vi "Display_data.vi"() -> ()   [LabVIEW 2016]
uses:
  <vilib>/Utility/file.llb/Read Delimited Spreadsheet (DBL).vi
panel:
  in  "Boolean":bool
  in  "STOP ALL":bool
  in  "stop":bool
  in  "Ring":u16(ring) items=["Default", "Number Filter", "Average", "Integrate", "Derivate", "g"]
  in  "String":string
  out "Waveform Graph 2":dbl[](graph)
  out "Array":dbl[](array[numeric])
  in  "X vector":i32
  out "XY Graph":cluster{dbl[], "all rows":dbl[]}[](graph)
  in  "Inoput":dbl=15.0 format="%#_13g"
  in  "index (row) 3":i32
  in  "index (row) 2":i32
  in  "index (row)":i32
  out "all rows":dbl[][](array[numeric])
  out "Raw Data":dynamicdata(graph)
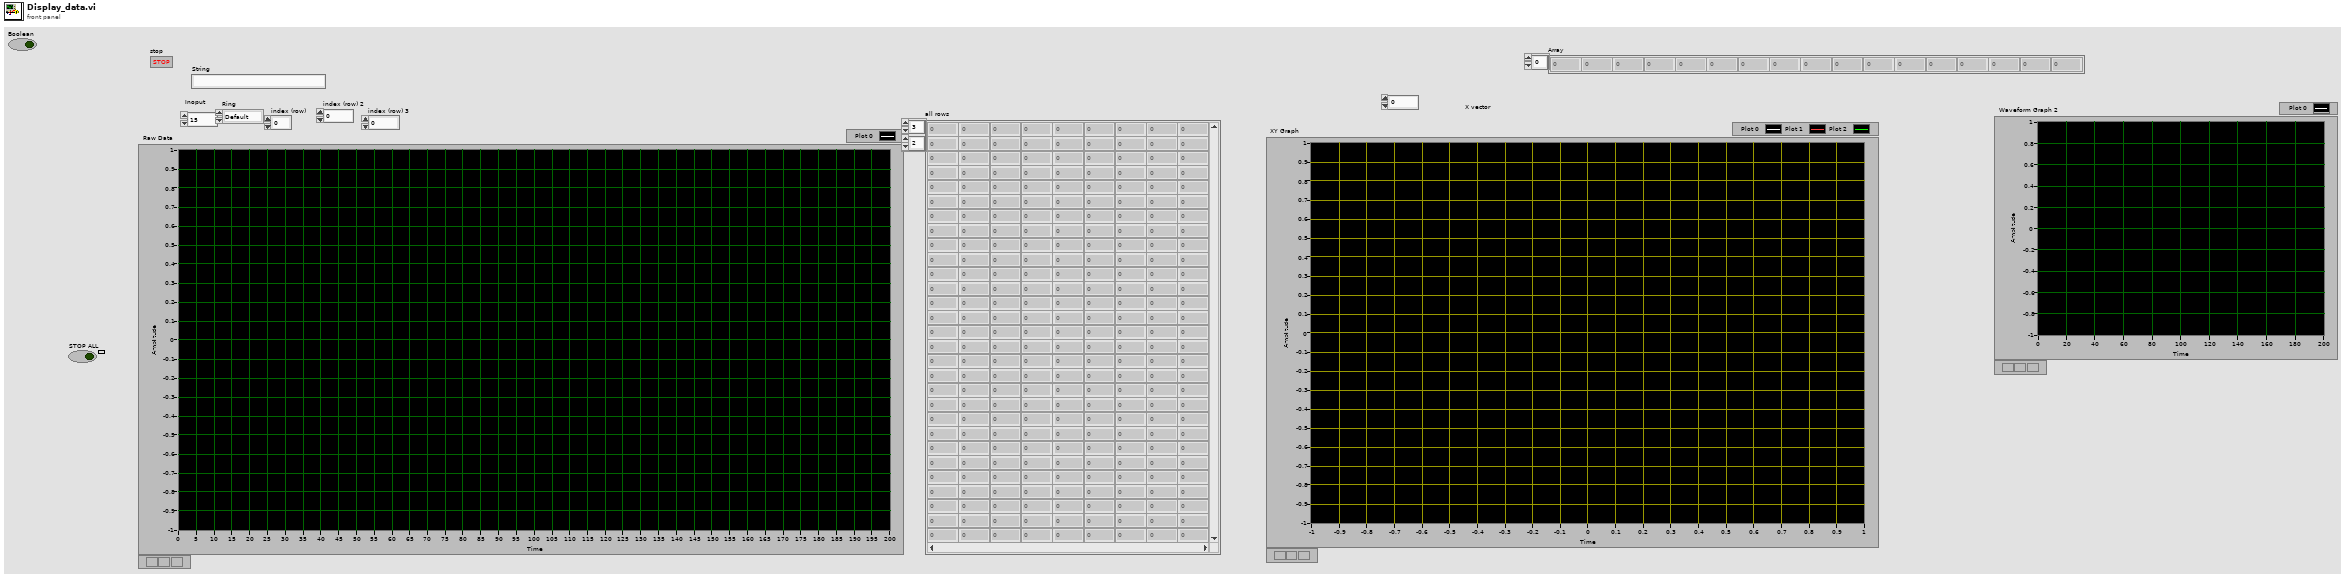
[diagram p1: front panel]
types:
  T1 = cluster{"Output Array":dbl[], "Output Array":dbl[]}
  T2 = cluster{"Output Array":dbl[], "Output Array":dbl[]}[]
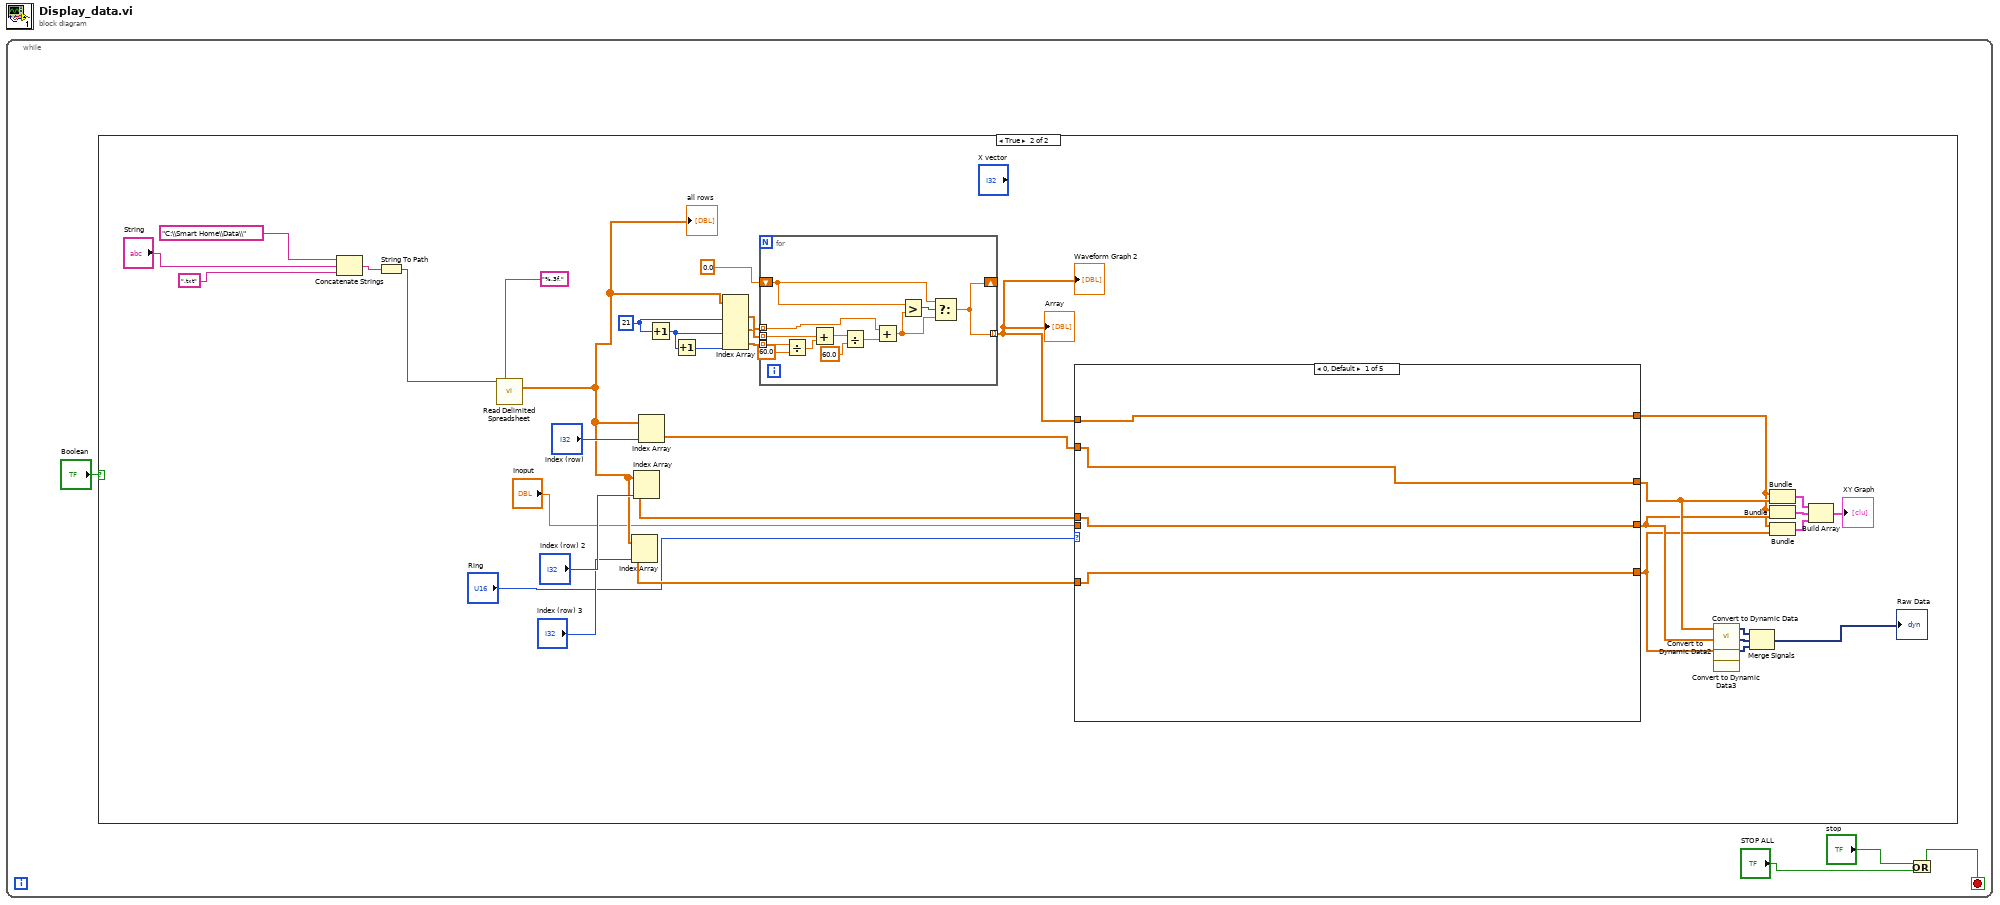
[diagram p0: block diagram]
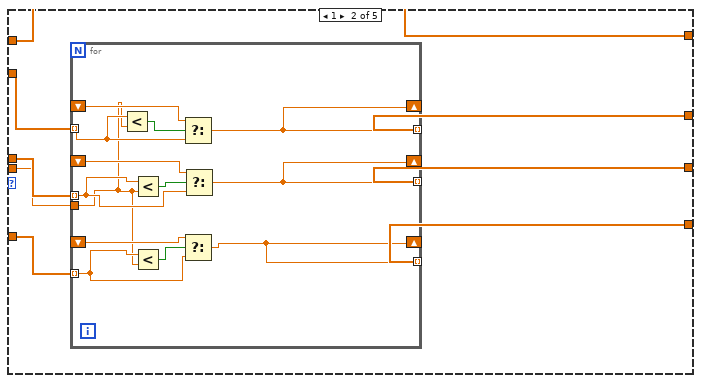
[diagram p3: hidden frame]
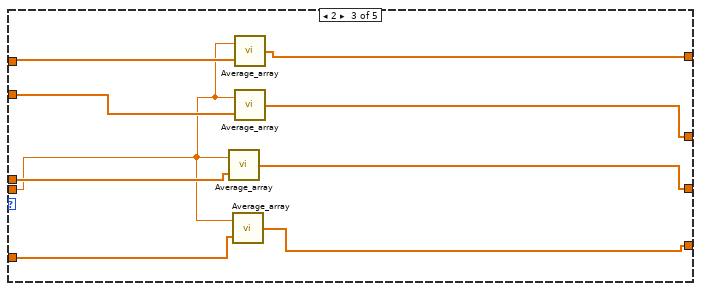
[diagram p4: hidden frame]
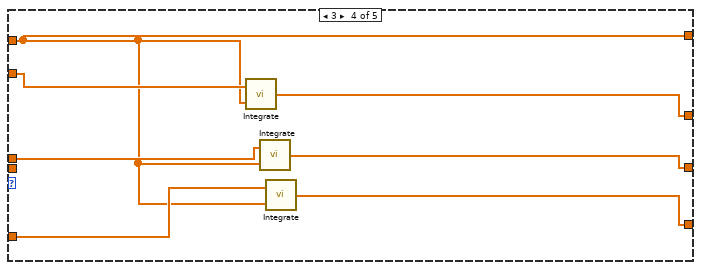
[diagram p5: hidden frame]
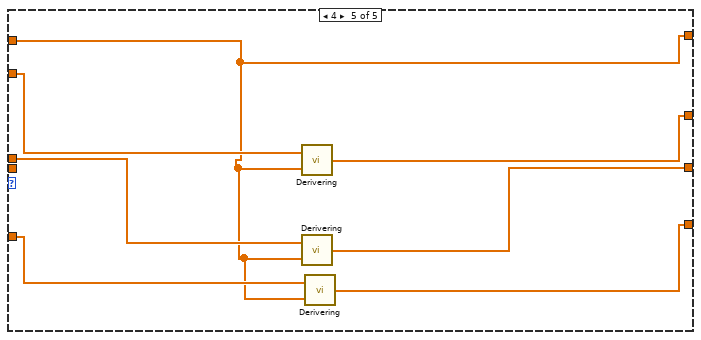
[diagram p6: hidden frame]
diagram:
  n1 = while {
    stop <- w3 stop-if-true
    n2 = case shown="True" "Boolean" {
      frame False {
      }
      frame True {
        w27 = 21 ("index (col)")
        n3 = Concatenate Strings("C:\\Smart Home\\Data\\", "String", ".txt") -> (w19:string)
        n4 = String To Path(string=w19) -> (path=w15:path)
        n5 = call-poly <vilib>:"Read Delimited Spreadsheet.vi"("file path (dialog if empty)"=w15, "format (%.3f)"="%.3f,") -> ("all rows"=w28:dbl[][])  [unwired: 8 in, 5 out]
        "all rows" <- w28
        n6 = Index Array(array=w28, index (col)="index (row) 3") -> (element=w29:dbl[])  [unwired: 1 in]
        n7 = Index Array(array=w28, index (col)="index (row) 2") -> (element=w30:dbl[])  [unwired: 1 in]
        n8 = Index Array(array=w28, index (col)="index (row)") -> (element=w31:dbl[])  [unwired: 1 in]
        n9 = Increment(x=w27) -> (x+1=w22:i32)
        n10 = Increment(x=w22) -> (x+1=w26:i32)
        n11 = Index Array(array=w28, index (col) #1=w27, index (col) #2=w22, index (col) #3=w26) -> (element #1=w25:dbl[], element #2=w24:dbl[], element #3=w23:dbl[])  [unwired: 3 in]
        n12 = for {
          tunnel: w25 -> [w43] mode=indexing
          tunnel: w24 -> [w45] mode=indexing
          tunnel: w23 -> [w44] mode=indexing
          tunnel: [w42] -> w6 mode=indexing
          shift-right: [w42] -> _
          shift-left: 0.0 -> [w41]
          n13 = Divide(x=w44, y=60.0) -> (x/y=w51:dbl)
          n14 = Add(x=w45, y=w51) -> (x+y=w46:dbl)
          n15 = Divide(x=w46, y=60.0) -> (x/y=w50:dbl)
          n16 = Add(x=w43, y=w50) -> (x+y=w40:dbl)
          n17 = Greater?(x=w41, y=w40) -> (0:w47:bool)
          n18 = Select(t=w41, s=w47, f=w40) -> (s? t:f=w42:dbl)
        }
        "Array" <- w6
        "Waveform Graph 2" <- w6
        n19 = case shown="0, Default" "Ring" {
          tunnel: w31 -> [w55 w63 w83 w90 w99]
          tunnel: w30 -> [w54 w62 w84 w91 w98]
          tunnel: w29 -> [w53 w61 w85 w92 w97]
          tunnel: [w53 w60 w80 w87 w96] -> w13
          tunnel: [w54 w59 w81 w88 w95] -> w14
          tunnel: [w55 w58 w82 w89 w94] -> w21
          tunnel: "Inoput" -> [_ w57 w78 _ _]
          tunnel: w6 -> [w52 w56 w79 w86 w93]
          tunnel: [w52 w56 w77 w86 w93] -> w5
          frame 0, Default {
          }
          frame 1 {
            n20 = for {
              tunnel: w63 -> [w74] mode=indexing
              tunnel: w62 -> [w71] mode=indexing
              tunnel: w61 -> [w68] mode=indexing
              shift-right: [w65] -> _
              shift-left: _ -> [w66]
              shift-right: [w70] -> _
              shift-left: _ -> [w69]
              shift-right: [w76] -> _
              shift-left: _ -> [w75]
              tunnel: [w76] -> w58 mode=indexing
              tunnel: [w70] -> w59 mode=indexing
              tunnel: [w65] -> w60 mode=indexing
              tunnel: w57 -> [w64]
              n21 = Less?(x=w74, y=w64) -> (x < y?=w73:bool)
              n22 = Less?(x=w71, y=w64) -> (x < y?=w72:bool)
              n23 = Less?(x=w68, y=w64) -> (x < y?=w67:bool)
              n24 = Select(t=w75, s=w73, f=w74) -> (s? t:f=w76:dbl)
              n25 = Select(t=w66, s=w67, f=w68) -> (s? t:f=w65:dbl)
              n26 = Select(t=w69, s=w72, f=w71) -> (s? t:f=w70:dbl)
            }
          }
          frame 2 {
            n27 = call "Average_array.vi"("Input Array"=w84, "Average over.."=w78) -> ("Output Array"=w81:dbl[])
            n28 = call "Average_array.vi"("Input Array"=w85, "Average over.."=w78) -> ("Output Array"=w80:dbl[])
            n29 = call "Average_array.vi"("Input Array"=w79, "Average over.."=w78) -> ("Output Array"=w77:dbl[])
            n30 = call "Average_array.vi"("Input Array"=w83, "Average over.."=w78) -> ("Output Array"=w82:dbl[])
          }
          frame 3 {
            n31 = call "Integrate.vi"("Input Array Y"=w86, "Input Array X"=w90) -> ("Output Array"=w89:dbl[])
            n32 = call "Integrate.vi"("Input Array Y"=w86, "Input Array X"=w91) -> ("Output Array"=w88:dbl[])
            n33 = call "Integrate.vi"("Input Array Y"=w86, "Input Array X"=w92) -> ("Output Array"=w87:dbl[])
          }
          frame 4 {
            n34 = call "Derivering.vi"("Input Array Y"=w93, "Input Array X"=w99) -> ("Output Array"=w94:dbl[])
            n35 = call "Derivering.vi"("Input Array Y"=w93, "Input Array X"=w98) -> ("Output Array"=w95:dbl[])
            n36 = call "Derivering.vi"("Input Array Y"=w93, "Input Array X"=w97) -> ("Output Array"=w96:dbl[])
          }
        }
        n37 = call "Convert to Dynamic Data"("Array"=w21) -> ("Dynamic Data Type"=w35:dynamicdata)  [unwired: 3 in]
        n38 = call "Convert to Dynamic Data2"("Array"=w14) -> ("Dynamic Data Type"=w34:dynamicdata)  [unwired: 3 in]
        n39 = call "Convert to Dynamic Data3"("Array"=w13) -> ("Dynamic Data Type"=w33:dynamicdata)  [unwired: 3 in]
        n40 = Merge Signals(w35, w34, w33) -> (→"Raw Data":dynamicdata)
        n41 = Bundle("Output Array"=w5, "Output Array"=w21) -> (w12:T1)  [unwired: 1 in]
        n42 = Bundle("Output Array"=w5, "Output Array"=w14) -> (w11:T1)  [unwired: 1 in]
        n43 = Bundle("Output Array"=w5, "Output Array"=w13) -> (w10:T1)  [unwired: 1 in]
        n44 = Build Array(w12, w11, w10) -> (→"XY Graph":T2)
      }
    }
    n45 = Or(x="stop", y="STOP ALL") -> (x .or. y?=w3:bool)
  }
